vi "TIO Avg AVM Field Data.vi"(8 "entrée d'erreur (pas d'erreur)":errorcluster, 10 "Component Index":i32, 11 "Tableau":T1(array[cluster])) -> (0 "sortie d'erreur":errorcluster, 4 "Total Average":dbl, 5 "dt":dbl, 7 "start":dbl)   [LabVIEW 2019]
panel:
  out "Total Data":dbl[](array[numeric])
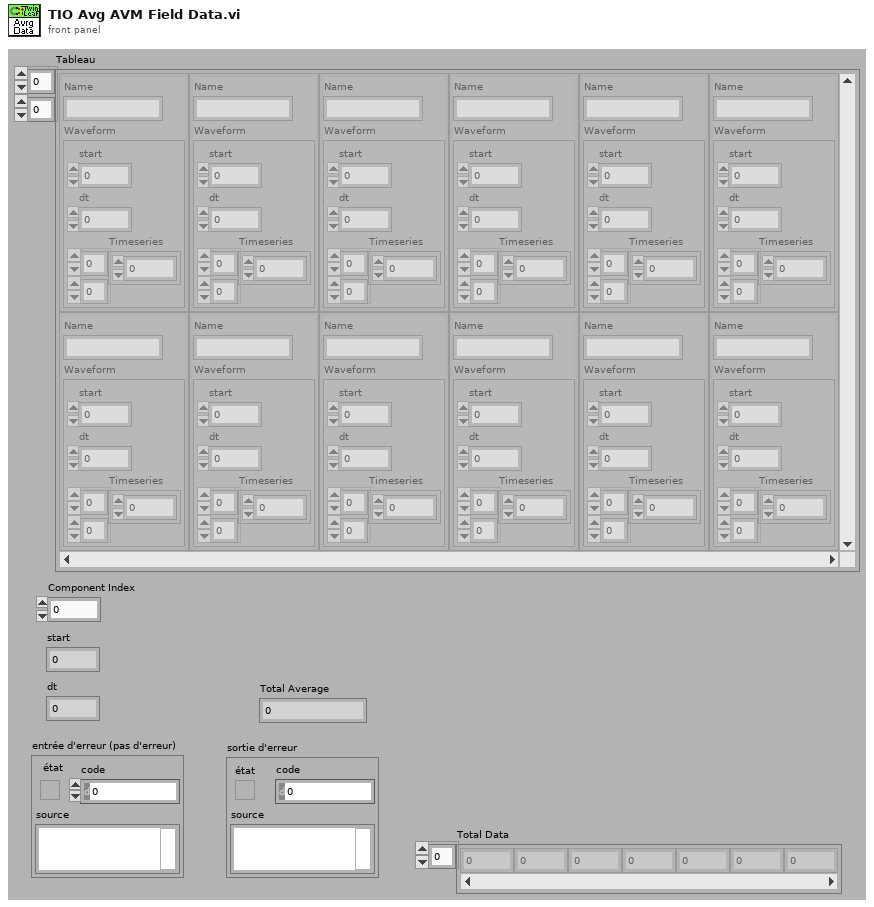
[diagram p1: front panel]
types:
  T1 = cluster{"Name":string, "Waveform":cluster{"start":dbl, "dt":dbl, "Timeseries":dbl[][]}}[][]
  T2 = cluster{"Name":string, "Waveform":cluster{"start":dbl, "dt":dbl, "Timeseries":dbl[][]}}
  T3 = cluster{"start":dbl, "dt":dbl, "Timeseries":dbl[][]}
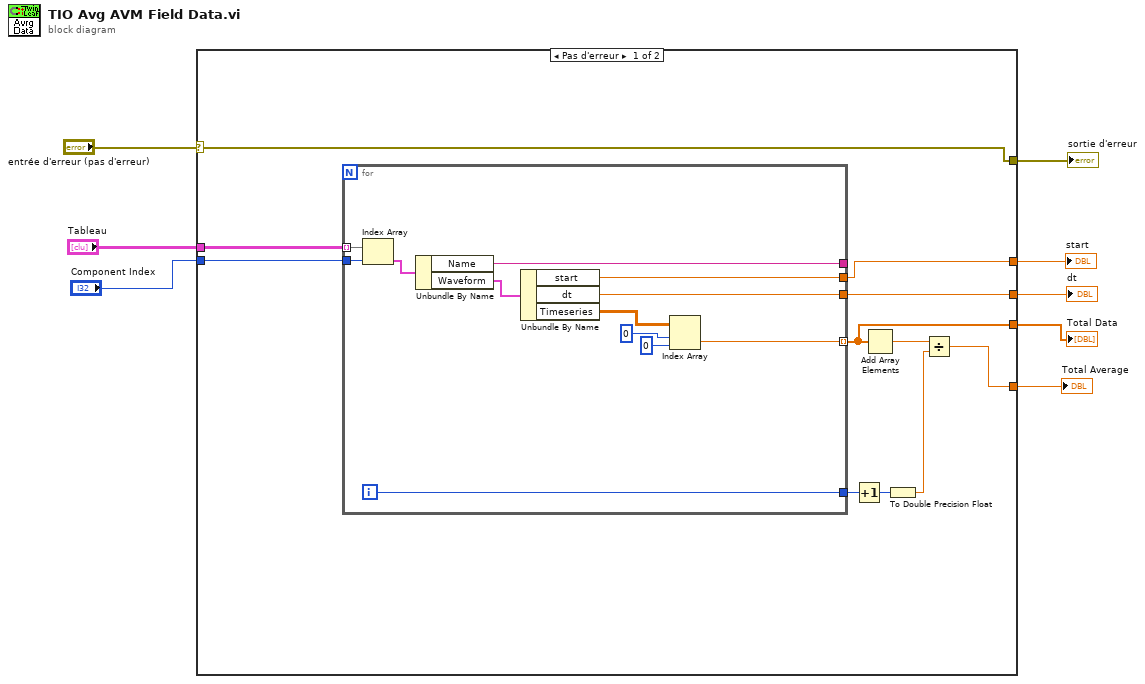
[diagram p0: block diagram]
diagram:
  n1 = case shown="Pas d'erreur" "entrée d'erreur (pas d'erreur)" {
    selector: "entrée d'erreur (pas d'erreur)" -> [w12 w32]
    tunnel: [w12 w32] -> w7
    tunnel: "Tableau" -> [w19 _]
    tunnel: "Component Index" -> [w18 _]
    tunnel: [w15 _] -> w4
    tunnel: [w14 _] -> w3
    tunnel: [w13 _] -> w1
    tunnel: [w10 _] -> w2
    frame No Error {
      n2 = for {
        tunnel: w19 -> [w31] mode=indexing
        tunnel: w18 -> [w29]
        tunnel: [w27] -> w15
        tunnel: [w26] -> w14
        tunnel: [w25] -> _
        tunnel: [w24] -> w16
        tunnel: [w20] -> w10 mode=indexing
        i -> [w24]
        n3 = Index Array(array=w31, index=w29) -> (element=w30:T2)
        n4 = Unbundle By Name(w30) -> ("Name"=w25:string, "Waveform"=w28:T3)
        n5 = Unbundle By Name(w28) -> ("start"=w27:dbl, "dt"=w26:dbl, "Timeseries"=w23:dbl[][])
        n6 = Index Array(array=w23, index (row)=0 ("indice désactivé (ligne)"), index (col)=0 ("indice désactivé (col)")) -> (element=w20:dbl)
      }
      n7 = Increment(x=w16) -> (x+1=w9:i32)
      n8 = Add Array Elements(numeric array=w10) -> (sum=w17:dbl)
      n9 = To Double Precision Float(number=w9) -> (double precision float=w11:dbl)
      n10 = Divide(x=w17, y=w11) -> (x/y=w13:dbl)
    }
    frame Error {
    }
  }
  "sortie d'erreur" <- w7
  "start" <- w4
  "dt" <- w3
  "Total Average" <- w1
  "Total Data" <- w2
